vi "Read Public Debug Terminal Events.vi"(8 "error in (no error)":errorcluster, 11 "DebuggingTerminal in":refnum<class "DebuggingTerminal.lvclass">) -> (0 "error out":errorcluster, 1 "Outgoing Stream":refnum<user-event>, 2 "Incoming Stream":refnum<user-event>, 3 "DebuggingTerminal out":refnum<class "DebuggingTerminal.lvclass">)   [LabVIEW 2013, in "MQTT Base.lvlib" / "DebuggingTerminal.lvclass"]
uses:
  DebuggingTerminal.lvclass
  DebuggingTerminal.lvclass/DebuggingTerminal.ctl
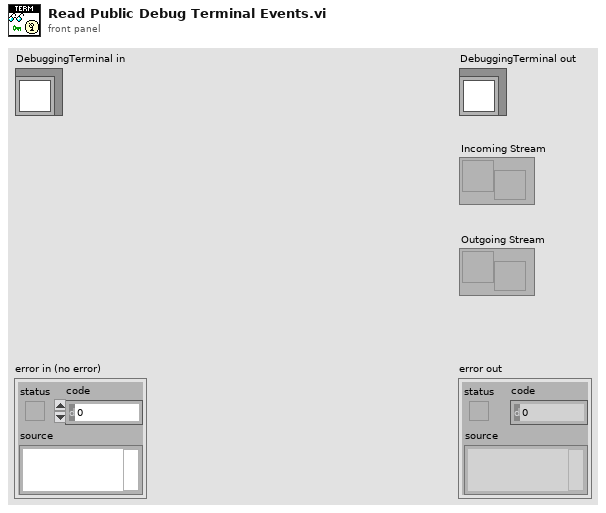
[diagram p1: front panel]
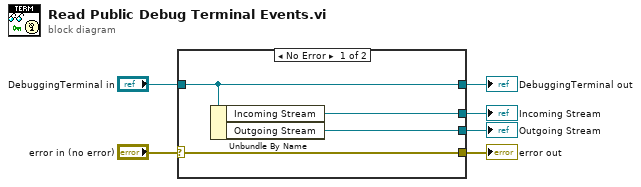
[diagram p0: block diagram]
diagram:
  n1 = case shown="No Error" "error in (no error)" {
    selector: "error in (no error)" -> [w10 w11]
    tunnel: [w10 w11] -> w5
    tunnel: [w9 w12] -> w3
    tunnel: "DebuggingTerminal in" -> [w9 w12]
    tunnel: [w8 _] -> w2
    tunnel: [w7 _] -> w1
    frame No Error {
      n2 = Unbundle By Name(w9) -> ("Incoming Stream"=w8:refnum<user-event>, "Outgoing Stream"=w7:refnum<user-event>)
    }
    frame Error {
    }
  }
  "error out" <- w5
  "DebuggingTerminal out" <- w3
  "Incoming Stream" <- w2
  "Outgoing Stream" <- w1
